vi "PicoLogHRDLExample.vi"() -> ()   [LabVIEW 2014]
uses:
  PicoHRDL.dll
panel:
  out "Meter":dbl(knob) scale=-2500.0..2500.0
  out "Over Voltage":i16
  out "Handle":i16
  in  "Single Ended":i16 min=0 max=1 step=1
  in  "Conversion":i16 min=0 max=5 step=1
  in  "Voltage Range":i16 min=0 max=6 step=1
  in  "Channel":i16=1 min=1 max=16 step=1
  # "-1        if the unit fails to open\n0         if no unit is found\n>= 1   handle to the device opened"
  # "The channel that will be enabled or disabled.\nADC-20: 1 to 8\nADC-24: 1 to 16"
  # "Non-zero to measure a single-ended voltage.\nZero for a differential voltage."
  # "range Voltage range Availability\n (0)    ±2500 mV        ADC-20 and ADC-24\n (1)    ±1250 mV        ADC-20 and ADC-24\n (2)    ±625 mV          ADC-24 only\n (3)    ±312.5 mV       ADC-24 only\n (4)    ±156.25 mV     ADC-24 only\n (5)    ±78.125 mV     ADC-24 only\n (6)    ±39.0625 mV   ADC-24 only"
  # "conversion Conversion time\n(0)               60 ms\n(1)               100 ms\n(2)               180 ms\n(3)               340 ms\n(4)               660 ms"
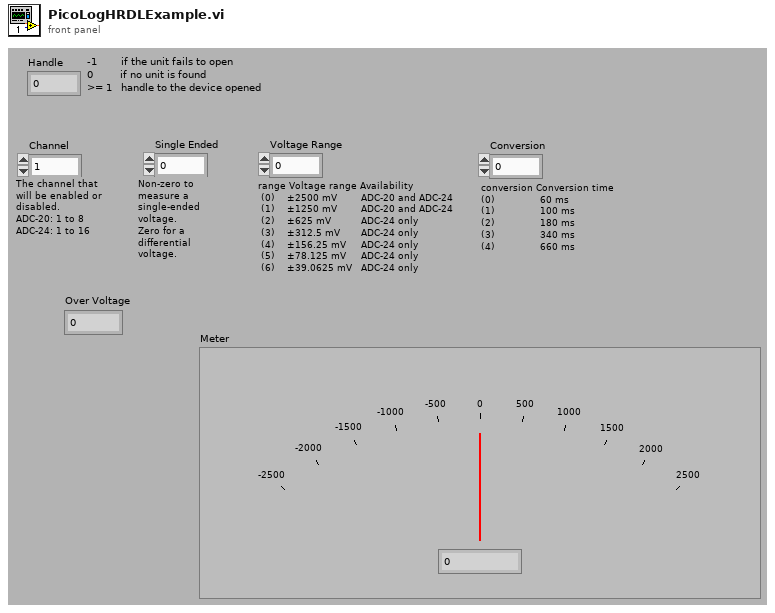
[diagram p1: front panel]
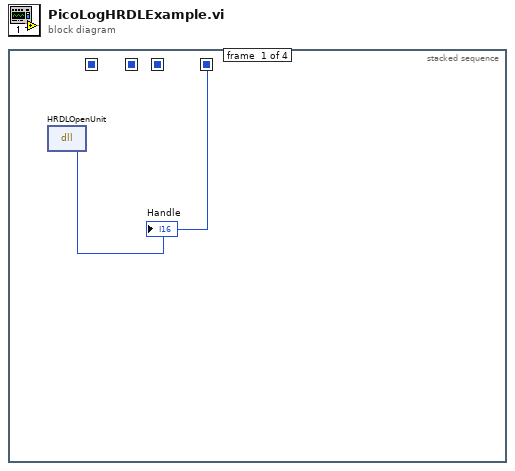
[diagram p0: block diagram]
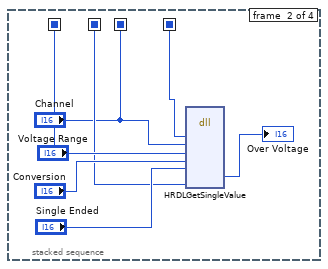
[diagram p2: hidden frame]
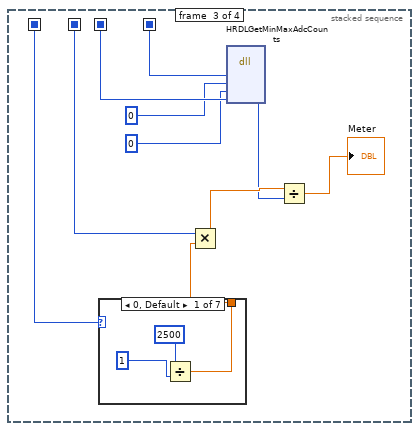
[diagram p3: hidden frame]
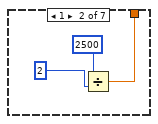
[diagram p4: hidden frame]
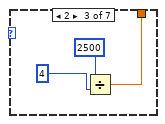
[diagram p5: hidden frame]
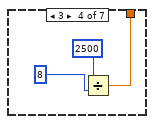
[diagram p6: hidden frame]
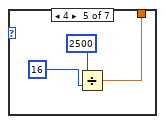
[diagram p7: hidden frame]
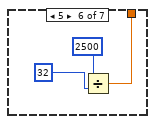
[diagram p8: hidden frame]
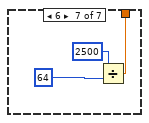
[diagram p9: hidden frame]
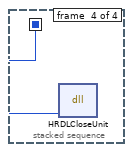
[diagram p10: hidden frame]
diagram:
  n1 = stacked-sequence {
    seq-local: [w1 _ _ _] -> [_ w6 w14 w40]
    seq-local: [_ "Voltage Range" _ _] -> [_ _ w18 _]
    seq-local: [_ w3 _ _] -> [_ _ w17 _]
    seq-local: [_ "Channel" _ _] -> [_ _ w13 _]
    frame #0 {
      n2 = dll-call lib="PicoHRDL.dll" fn="HRDLOpenUnit"() -> (w1:i16)  [unwired: 3 in, 2 out]
      "Handle" <- w1
    }
    frame #1 {
      n3 = dll-call lib="PicoHRDL.dll" fn="HRDLGetSingleValue"("handle"=w6, "channel"="Channel", "range"="Voltage Range", "conversionTime"="Conversion", "singleEnded"="Single Ended") -> ("overflow"=→"Over Voltage":i16, "value"=w3:i16)  [unwired: 11 in, 2 out]
    }
    frame #2 {
      n4 = case shown="0, Default" w18 {
        tunnel: [w19 w22 w25 w28 w31 w34 w37] -> w16
        frame 0, Default {
          n5 = Divide(x=2500, y=1) -> (x/y=w19:dbl)
        }
        frame 1 {
          n6 = Divide(x=2500, y=2) -> (x/y=w22:dbl)
        }
        frame 2 {
          n7 = Divide(x=2500, y=4) -> (x/y=w25:dbl)
        }
        frame 3 {
          n8 = Divide(x=2500, y=8) -> (x/y=w28:dbl)
        }
        frame 4 {
          n9 = Divide(x=2500, y=16) -> (x/y=w31:dbl)
        }
        frame 5 {
          n10 = Divide(x=2500, y=32) -> (x/y=w34:dbl)
        }
        frame 6 {
          n11 = Divide(x=2500, y=64) -> (x/y=w37:dbl)
        }
      }
      n12 = Multiply(x=w17, y=w16) -> (x*y=w15:dbl)
      n13 = dll-call lib="PicoHRDL.dll" fn="HRDLGetMinMaxAdcCounts"("handle"=w14, "minAdc"=0, "maxAdc"=0, "channel"=w13) -> ("maxAdc"=w12:i32)  [unwired: 7 in, 2 out]
      n14 = Divide(x=w15, y=w12) -> (x/y=→"Meter":dbl)
    }
    frame #3 {
      n15 = dll-call lib="PicoHRDL.dll" fn="HRDLCloseUnit"("handle"=w40) -> ()  [unwired: 5 in, 2 out]
    }
  }
